vi "m1m3_logEvent_HardpointMonitorState.vi"(8 "error in (no error)":errorcluster, 11 "logevent_HardpointMonitorState_Ctl":T1={"Timestamp"=0.0, "ILCState[6]"=[0, 0, 0, 0, 0, 0], "priority"=0}) -> (0 "error out":errorcluster, 2 "function return":i32, 3 "logevent_HardpointMonitorState_Ctl out":T1)   [LabVIEW 2016, in "SALLV_m1m3.lvlib"]
doc: "int m1m3_shm_logEvent_HardpointMonitorStateLV(m1m3_logevent_HardpointMonitorStateLV *logevent_HardpointMonitorState_Ctl );"
uses:
  SALLV_m1m3.lvlib
  DataTypes/logevent_HardpointMonitorState.ctl
  SALLV_m1m3.so
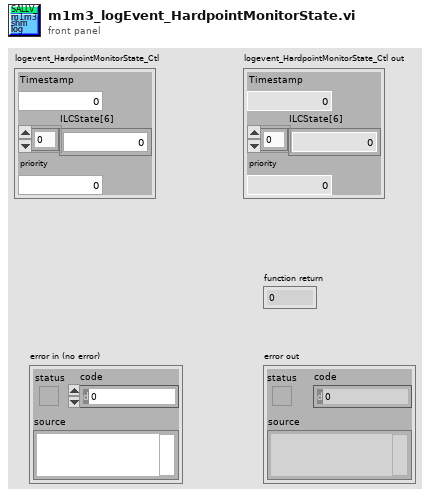
[diagram p1: front panel]
types:
  T1 = typedef "SALLV_m1m3.lvlib/logevent_HardpointMonitorState.ctl" = cluster{"Timestamp":dbl, "ILCState[6]":i16[], "priority":i32}
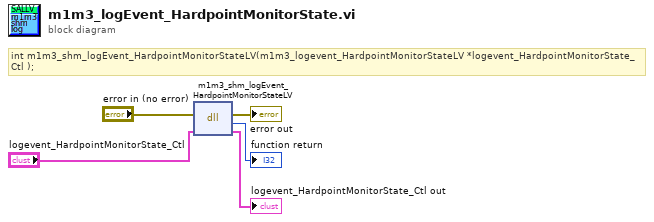
[diagram p0: block diagram]
diagram:
  # "int m1m3_shm_logEvent_HardpointMonitorStateLV(m1m3_logevent_HardpointMonitorStateLV *logevent_HardpointMonitorState_Ctl );"
  n1 = dll-call lib="opt/CODE/SALLV_m1m3/SALLV_m1m3.*" fn="m1m3_shm_logEvent_HardpointMonitorStateLV"(error in="error in (no error)", "logevent_HardpointMonitorState_Ctl"="logevent_HardpointMonitorState_Ctl") -> (error out=→"error out":errorcluster, →"function return":i32, "logevent_HardpointMonitorState_Ctl"=→"logevent_HardpointMonitorState_Ctl out":T1)  [unwired: 2 in, 1 out]
